vi "Get Array Index Combo Box.vi"(8 "error in (no error)":errorcluster, 11 "Array in":refnum<vi>) -> (0 "error out":errorcluster, 2 "ComboBox out":refnum<vi>)   [LabVIEW 2016]
doc: "Looks at the array of clusters and finds the reference to the combo box inside the elements type definition"
uses:
  Assert Build Configuration.ctl
  Core/Assert API Components/Failure Actions.ctl
  Core/Assert API Components/Assert API Components.lvlib
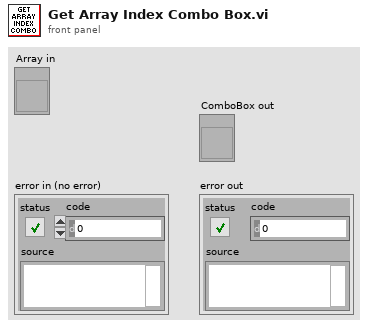
[diagram p1: front panel]
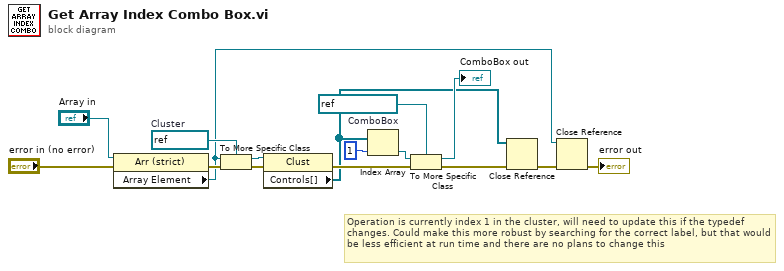
[diagram p0: block diagram]
diagram:
  w9 = refnum<vi> refnum  # Cluster
  w6 = refnum<vi> refnum  # ComboBox
  # "Operation is currently index 1 in the cluster, will need to update this if the typedef changes. Could make this more robust by searching for the correct label, but that would be less efficient at run time and there are no plans to change this"
  n1 = property class="Arr (strict)"(reference="Array in", error in="error in (no error)") -> (error out=w15:errorcluster, "Array Element"=w2:refnum<vi>)  [unwired: 1 out]
  n2 = To More Specific Class(target class=w9, reference=w2, error in=w15) -> (specific class reference=w10:refnum<vi>, error out=w11:errorcluster)
  n3 = property class="Clust"(reference=w10, error in=w11) -> (error out=w14:errorcluster, "Controls[]"=w4:refnum<vi>[])  [unwired: 1 out]
  n4 = Index Array(array=w4, index=1) -> (element=w13:refnum<vi>)
  n5 = To More Specific Class(target class=w6, reference=w13, error in=w14) -> (specific class reference=→"ComboBox out":refnum<vi>, error out=w1:errorcluster)
  n6 = Close Reference(reference=w4, error in (no error)=w1) -> (error out=w5:errorcluster)
  n7 = Close Reference(reference=w2, error in (no error)=w5) -> (error out=→"error out":errorcluster)
